vi "PDA test.vi"() -> ()   [LabVIEW 2020]
uses:
  <vilib>/Analysis/NI_AALBase.lvlib
panel:
  out "Waveform Graph 2":dbl[](graph)
  in  "Subtract Bg":bool
  in  "SaveBg":bool
  in  "stop":bool
  out "standard deviation":dbl format="%0.2f"
  out "Waveform Chart":dbl[](graph)
  out "Waveform Graph":dbl[][](graph)
  in  "Shutter Mode":bool
  in  "Number of Accumulations":i16=5
  out "error out":errorcluster
  out "Avg value":dbl format="%0.2f"
  out "Final Data Array":dbl[](array[numeric]) format="%.2f"
  in  "error in":errorcluster
  in  "StartIng Mode":T1(ring)
  in  "Acquisition Parameters":T2={"Exposure (ms)"=100, "Interval (ms)"=100, "Flush Count"=1, "Trigger"=0} {"Trigger" items=["Disable", "Acquistion", "Cycle"]}
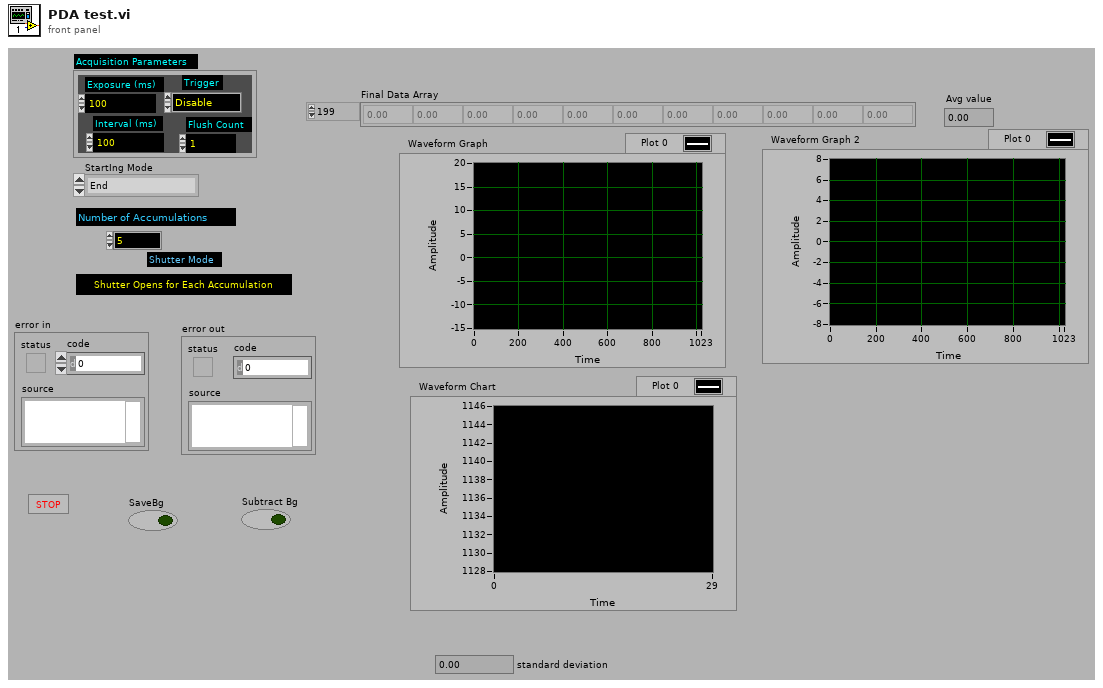
[diagram p1: front panel]
types:
  T1 = enum16{"End", "Init", "Reset", "SetAcqParameter", "SetArea", "AcqData"}
  T2 = cluster{"Exposure (ms)":u32, "Interval (ms)":u32, "Flush Count":i32, "Trigger":u16}
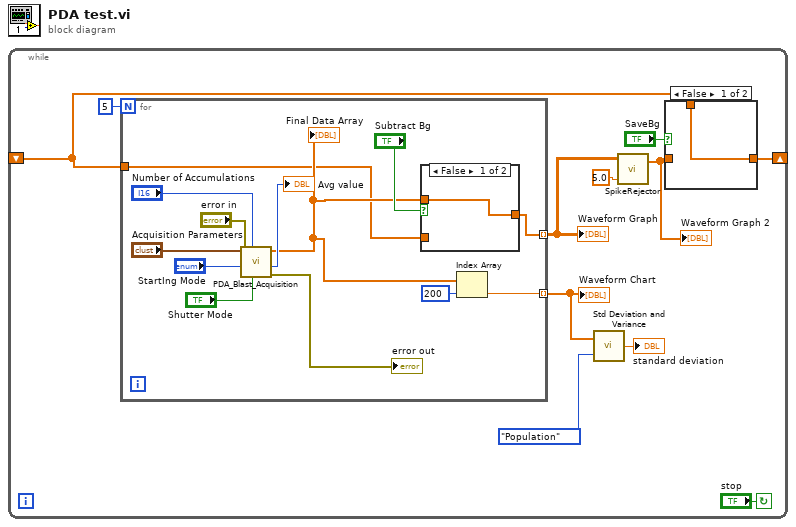
[diagram p0: block diagram]
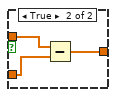
[diagram p3: hidden frame]
diagram:
  n1 = while {
    shift-right: [w3] -> _
    shift-left: _ -> [w2]
    stop <- "stop" continue-if-true
    n2 = for {
      N: 5 -> [_]
      tunnel: [w14] -> w6 mode=indexing
      tunnel: [w18] -> w10 mode=indexing
      tunnel: w2 -> [w15]
      n3 = call "PDA_Blast_Acquisition.vi"("Shutter Mode"="Shutter Mode", "Number of Accumulations"="Number of Accumulations", "error in"="error in", "StartIng Mode"="StartIng Mode", "Acquisition Parameters"="Acquisition Parameters") -> ("error out"=→"error out":errorcluster, "Pixel Overflow"=→"Avg value":i32, "Final Data Array"=w16:dbl[])  [unwired: 1 in, 1 out]
      "Final Data Array" <- w16
      n4 = case shown="False" "Subtract Bg" {
        tunnel: w16 -> [w27 w30]
        tunnel: w15 -> [_ w29]
        tunnel: [w27 w28] -> w14
        frame False {
        }
        frame True {
          n5 = Subtract(x=w30, y=w29) -> (x-y=w28:dbl[])
        }
      }
      n6 = Index Array(array=w16, index=200) -> (element=w18:dbl)
    }
    "Waveform Graph" <- w6
    "Waveform Chart" <- w10
    n7 = call <vilib>:"Std Deviation and Variance.vi"("X"=w10, "Weighting (Sample)"=enum16{"Sample", "Population"}."Population") -> ("standard deviation"=→"standard deviation":dbl)  [unwired: 2 out]
    n8 = call "SpikeRejector.vi"("SigmaFactor"=5.0, "Input Array"=w6) -> ("Final Array"=w1:dbl[])  [unwired: 2 in, 1 out]
    "Waveform Graph 2" <- w1
    n9 = case shown="False" "SaveBg" {
      tunnel: [w12 w13] -> w3
      tunnel: w1 -> [_ w13]
      tunnel: w2 -> [w12 _]
      frame False {
      }
      frame True {
      }
    }
  }
